vi "Untitled 1.vi"() -> ()   [LabVIEW 2019]
uses:
  <vilib>/Instr/_visa.llb/VISA Configure Serial Port (Instr).vi
panel:
  out "Waveform Chart":dbl(graph)
  out "Numeric":dbl
  in  "stop":bool
  out "number of iteration":i32
  out "read buffer":string
  out "return count":u32
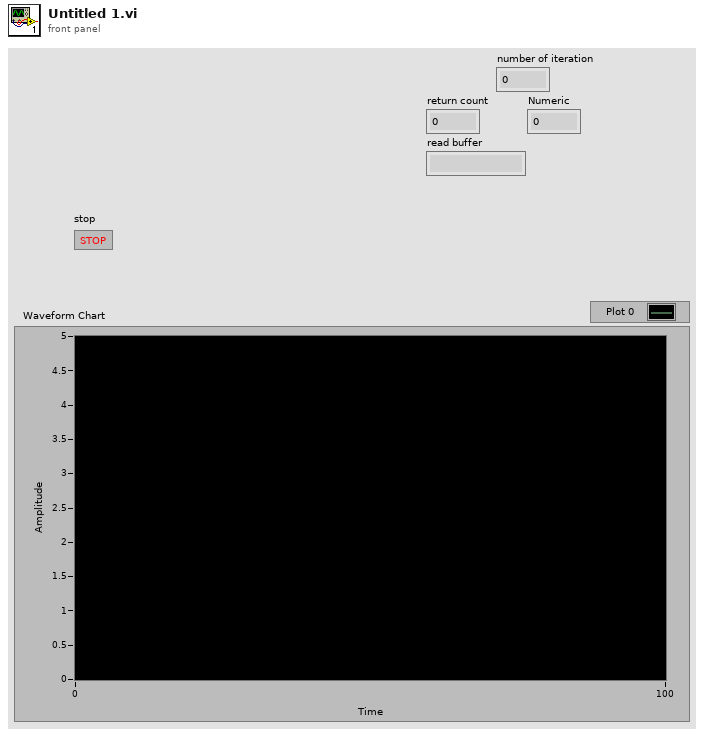
[diagram p1: front panel]
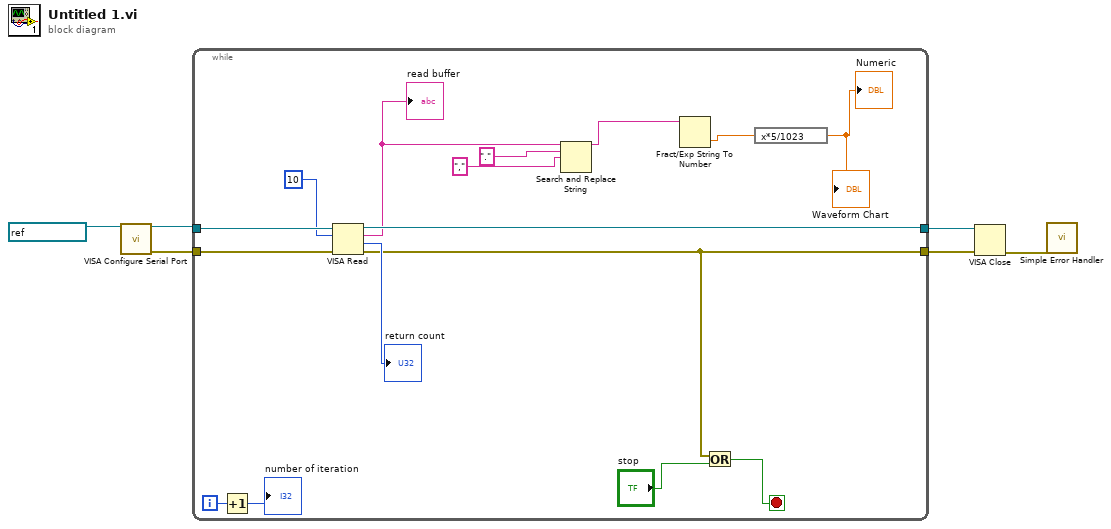
[diagram p0: block diagram]
diagram:
  n1 = call-poly "VISA Configure Serial Port"("VISA resource name"=refnum<visa-resource-name> "COM4") -> ("VISA resource name out"=w5:refnum<visa-resource-name>, "error out"=w4:errorcluster)  [unwired: 13 in]
  n2 = while {
    tunnel: w5 -> [w22]
    tunnel: [w19] -> w3
    tunnel: w4 -> [w21]
    tunnel: [w15] -> w2
    i -> [w17]
    stop <- w13 stop-if-true
    n3 = Increment(x=w17) -> (x+1=→"number of iteration":i32)
    n4 = VISA Read(VISA resource name=w22, byte count=u32 10, error in (no error)=w21) -> (VISA resource name out=w19:refnum<visa-resource-name>, read buffer=w12:string, return count=→"return count":u32, error out=w15:errorcluster)
    "read buffer" <- w12
    n5 = Search and Replace String(input string=w12, search string=".", replace string="," ("replace string (\"\")")) -> (result string=w10:string)  [unwired: 5 in, 3 out]
    n6 = Fract/Exp String To Number(string=w10) -> (number=w8:dbl)  [unwired: 3 in, 1 out]
    n7 = Or(x=w15, y="stop") -> (x .or. y?=w13:bool)
    n8 = expression code="x*5/1023"(w8) -> (→"Numeric" →"Waveform Chart":dbl)
  }
  n9 = VISA Close(VISA resource name=w3, error in (no error)=w2) -> (error out=w1:errorcluster)
  n10 = call <vilib>:"Simple Error Handler.vi"("error in (no error)"=w1) -> ()  [unwired: 4 in, 5 out]
